vi "WPI_CameraAcquire JPG Loop.vi"(11 "CameraDevRef":T1) -> ()   [LabVIEW 2017]
doc: "This VI acquires the image buffer from the camera JPG stream at the configured fps rate. It notifies any waiting VIs and allows them to pick up the latest image. This allows the camera and robot vision loop to run at different rates. This loop times the camera images from the cRIO, and tends to minimize latency, but with the 1011 camera, the overhead of the JPG requests is quite high, and the MJPG loop is far more efficient.\n\nThis software is licensed. Open the labview\\readme\\WPI Robotics Library Open Source License.txt file for more information."
uses:
  <vilib>/Rock Robotics/WPI/Camera/WPI_CameraDevRef.ctl
  <vilib>/Rock Robotics/WPI/Camera/WPI_CameraSettings Operations.ctl
  <vilib>/Rock Robotics/WPI/Camera/WPI_CameraFrameRate.ctl
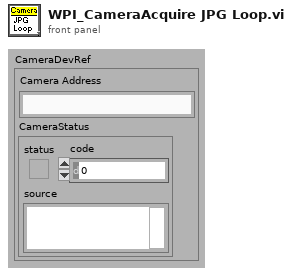
[diagram p1: front panel]
types:
  T1 = typedef "WPI_CameraDevRef.ctl" = cluster{"Camera Address":string, "CameraStatus":errorcluster}
  T2 = typedef "WPI_CameraSettings Operations.ctl" = enum16{"Udate FPS", "Update Compression", "Update Size", "Update White Balance", "Update Brightness", "Update Sharpness", "Update Exposure", "Update Exposure Value", "Update Color Level", "Update Exp Priority", "Update Color Enable", "Update JPG", "Update MJPG", "Read and Clear", "Read", "Init"}
  T3 = typedef "WPI_CameraFrameRate.ctl" = u32
  T4 = typedef "WPI_CameraSettings Control.ctl" = cluster{"FPS":i32, "Compression":i32, "Size":i32, "White Balance":i32, "Brightness":i32, "Sharpness":i32, "Exposure":i32, "Color Level":i32, "Exposure Priority":i32, "Color Enable":i32, "JPG Loop":i32, "MJPG Loop":i32, "Exposure Value":i32}
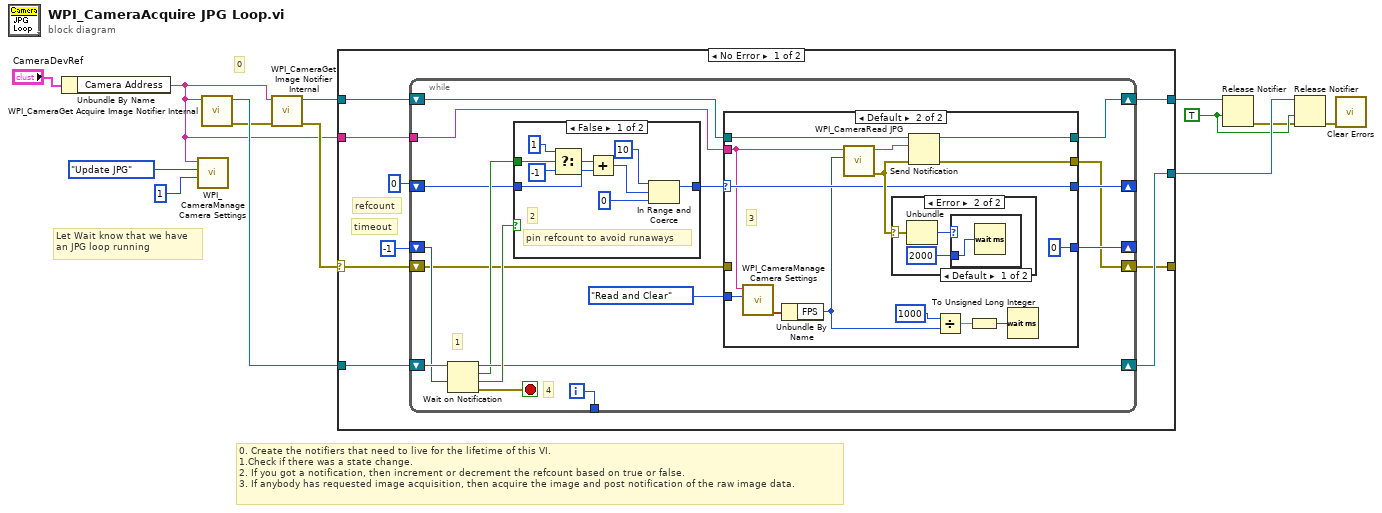
[diagram p0: block diagram]
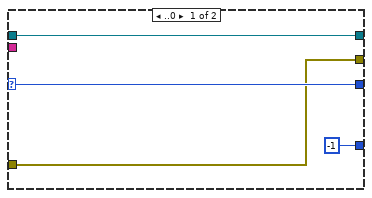
[diagram p2: hidden frame]
diagram:
  w10 = TRUE ("force destroy? (F)")
  # "Let Wait know that we have\nan JPG loop running"
  # "0"
  # "0. Create the notifiers that need to live for the lifetime of this VI. \n1.Check if there was a state change.\n2. If you got a notification, then increment or decrement the refcount based on true or false.\n3. If anybody has requested image acquisition, then acquire the image and post notification of the raw image data."
  n1 = Unbundle By Name("CameraDevRef") -> ("Camera Address"=w1:string)
  n2 = call <vilib>:"WPI_CameraManage Camera Settings.vi"("Value"=1, "Operation"=WPI_CameraSettings_Operations."Update JPG", "Camera IP"=w1) -> ()  [unwired: 7 in, 2 out]
  n3 = call <vilib>:"WPI_CameraGet Acquire Image Notifier Internal.vi"("Camera Address"=w1) -> ("error out"=w5:errorcluster, "Acquire Image Notifier"=w6:refnum<notifier>)  [unwired: 1 in, 8 out]
  n4 = call <vilib>:"WPI_CameraGet Image Notifier Internal.vi"("error in (no error)"=w5, "Camera Address"=w1) -> ("error out"=w8:errorcluster, "Image Notifier"=w11:refnum<notifier>)  [unwired: 8 out]
  n5 = case shown="No Error" w8 {
    selector: w8 -> [w15 w74]
    tunnel: w1 -> [w22 _]
    tunnel: w6 -> [w21 w72]
    tunnel: w11 -> [w19 w73]
    tunnel: [w17 w73] -> w13
    tunnel: [w16 w72] -> w12
    tunnel: [w14 w74] -> _
    frame No Error {
      # "timeout"
      # "refcount"
      n6 = while {
        shift-right: [w37] -> w16
        shift-left: w21 -> [w39]
        tunnel: w22 -> [w34]
        shift-right: [w26] -> _
        shift-left: 0 -> [w35]
        shift-right: [w32] -> w17
        shift-left: w19 -> [w33]
        shift-right: [w30] -> _
        shift-left: -1 -> [w31]
        shift-right: [w25] -> w14
        shift-left: w15 -> [w28]
        tunnel: [w23] -> _
        i -> [w23]
        stop <- w29 stop-if-true
        # "4"
        # "1"
        n7 = Wait on Notification(notifier=w39, timeout in ms (-1)=w31) -> (notifier out=w37:refnum<notifier>, notification=w36:bool, timed out?=w38:bool, error out=w29:errorcluster)  [unwired: 1 in, 1 out]
        n8 = case shown="False" w38 {
          tunnel: w36 -> [w70 _]
          tunnel: w35 -> [w66 w71]
          tunnel: [w62 w71] -> w27
          frame False {
            # "pin refcount to avoid runaways"
            # "2"
            n9 = Select(t=1, s=w70, f=-1) -> (s? t:f=w67:i32)
            n10 = Add(x=w67, y=w66) -> (x+y=w63:i32)
            n11 = In Range and Coerce(upper limit=10, x=w63, lower limit=0) -> (coerced(x)=w62:i32)  [unwired: 1 out]
          }
          frame True {
          }
        }
        n12 = case shown="Default" w27 {
          selector: w27 -> [w42 w52]
          tunnel: w34 -> [_ w44]
          tunnel: w33 -> [w43 w57]
          tunnel: [w43 w56] -> w32
          tunnel: [-1 0] -> w30
          tunnel: w28 -> [w40 _]
          tunnel: [w42 w52] -> w26
          tunnel: [w40 w48] -> w25
          tunnel: WPI_CameraSettings_Operations."Read and Clear" ("Operation") -> [_ w47]
          frame ..0 {
          }
          frame Default {
            # "3"
            n13 = call <vilib>:"WPI_CameraManage Camera Settings.vi"("Operation"=w47, "Camera IP"=w44) -> ("Values"=w46:T4)  [unwired: 8 in, 1 out]
            n14 = Unbundle By Name(w46) -> ("FPS"=w45:i32)
            n15 = call <vilib>:"WPI_CameraRead JPG.vi"("fps"=w45, "address"=w44) -> ("error out"=w53:errorcluster, "Raw Image Data"=w54:string)  [unwired: 2 in, 6 out]
            n16 = case shown="Error" w53 {
              selector: w53 -> [_ w60]
              frame No Error {
              }
              frame Error {
                n17 = Unbundle(w60) -> ("code"=w59:i32)  [unwired: 2 out]
                n18 = case shown="Default" w59 {
                  tunnel: u32 2000 ("milliseconds to wait") -> [w61 _]
                  frame Default {
                    n19 = Wait (ms)(milliseconds to wait=w61) -> ()  [unwired: 1 out]
                  }
                  frame 56 {
                  }
                }
              }
            }
            n20 = Send Notification(notification=w54, notifier=w57, error in (no error)=w53) -> (notifier out=w56:refnum<notifier>, error out=w48:errorcluster)
            n21 = Divide(x=T3 1000, y=w45) -> (x/y=w50:dbl)
            n22 = To Unsigned Long Integer(number=w50) -> (unsigned 32bit integer=w51:u32)
            n23 = Wait (ms)(milliseconds to wait=w51) -> ()  [unwired: 1 out]
          }
        }
      }
    }
    frame Error {
    }
  }
  n24 = Release Notifier(notifier=w13, force destroy? (F)=w10) -> (error out=w4:errorcluster)  [unwired: 1 in, 2 out]
  n25 = Release Notifier(notifier=w12, force destroy? (F)=w10, error in (no error)=w4) -> (error out=w7:errorcluster)  [unwired: 2 out]
  n26 = call <vilib>:"Clear Errors.vi"("error in (no error)"=w7) -> ()  [unwired: 1 in, 6 out]
